vi "GSP_Manager_SCLNClient_Handler.vi"(4 "error in (no error)":errorcluster, 6 "Actions":T1) -> (0 "error out":errorcluster, 2 "reference out (launch only)":refnum<vi>)   [LabVIEW 2015]
uses:
  TCS_Link/TCSLINK_handler_actions.ctl
panel:
  out "Config filename":path=path "examples.cfg"
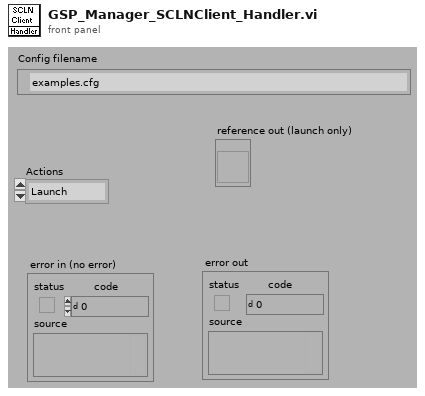
[diagram p1: front panel]
types:
  T1 = typedef "TCSLINK_handler_actions.ctl" = enum16{"Launch", "Shutdown"}
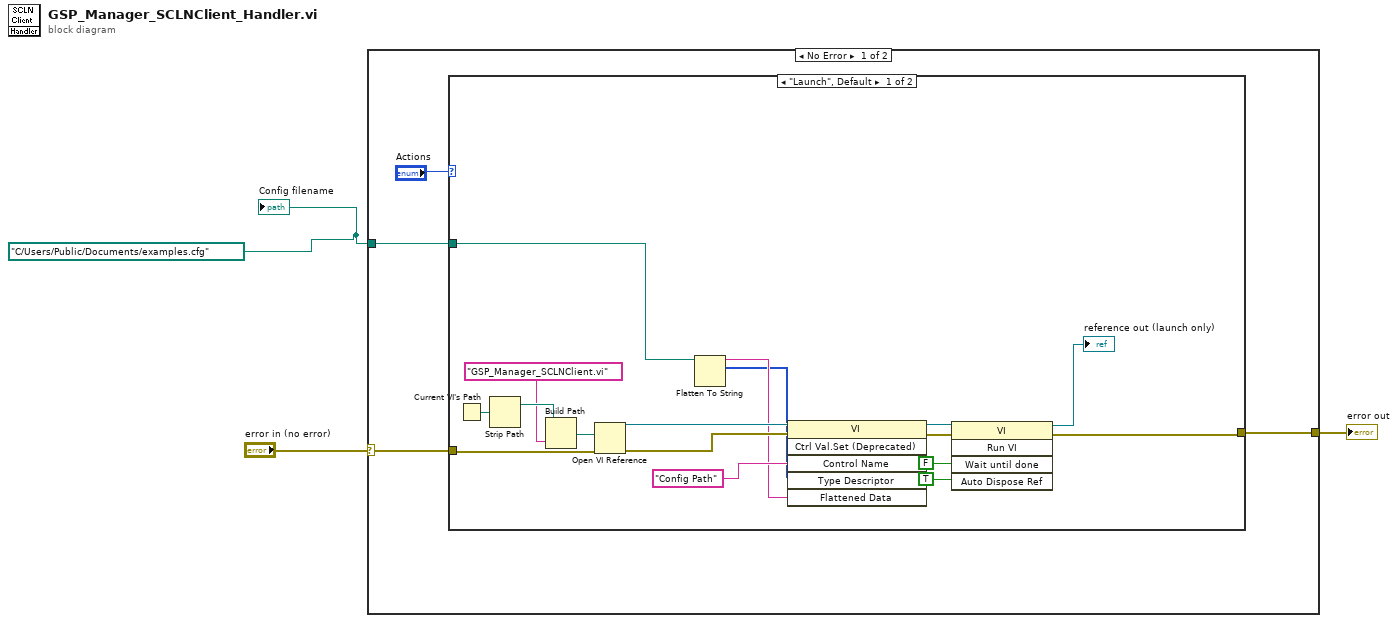
[diagram p0: block diagram]
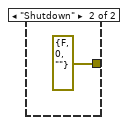
[diagram p2: hidden frame]
diagram:
  w1 = path "C:/Users/Public/Documents/examples.cfg"
  n1 = case shown="No Error" "error in (no error)" {
    selector: "error in (no error)" -> [w6 w26]
    tunnel: [w7 w26] -> w3
    tunnel: w1 -> [w4 _]
    frame No Error {
      n2 = case shown="\"Launch\", Default" "Actions" {
        tunnel: w6 -> [w24 _]
        tunnel: [w17 errorcluster {"status"=FALSE, "code"=0, "source"=""} ("error out")] -> w7
        tunnel: w4 -> [w8 _]
        frame "Launch", Default {
          n3 = Current VI's Path() -> (path=w21:path)
          n4 = Strip Path(path=w21) -> (stripped path=w19:path)  [unwired: 1 out]
          n5 = Build Path(base path=w19, name or relative path="GSP_Manager_SCLNClient.vi" ("vi path")) -> (appended path=w20:path)
          n6 = Open VI Reference(vi path=w20, error in (no error)=w24) -> (vi reference=w13:refnum<vi>, error out=w12:errorcluster)  [unwired: 4 in]
          n7 = Flatten To String(anything=w8) -> (data string=w10:string, type string=w9:i16[])  [unwired: 3 in, 1 out]
          n8 = invoke class="VI" method="Ctrl Val.Set (Deprecated)"(reference=w13, error in=w12, "Control Name"="Config Path", "Type Descriptor"=w9, "Flattened Data"=w10) -> (reference out=w15:refnum<vi>, error out=w14:errorcluster)  [unwired: 1 in, 4 out]
          n9 = invoke class="VI" method="Run VI"(reference=w15, error in=w14, "Wait until done"=FALSE, "Auto Dispose Ref"=TRUE) -> (reference out=→"reference out (launch only)":refnum<vi>, error out=w17:errorcluster)  [unwired: 1 in, 3 out]
        }
        frame "Shutdown" {
        }
      }
    }
    frame Error {
    }
  }
  "error out" <- w3
  "Config filename" <- w1
